vi "PDash - Create DQMH Module Template.vi"(11 "Template Folder":path) -> (0 "error out":errorcluster)   [LabVIEW 2020]
doc: "_____\nCreated using DQMH Event Scripter 7.1.0.1447."
uses:
  PantherDashboard Scripting Hooks/Panther Dasboard Scripting Hooks.lvlib
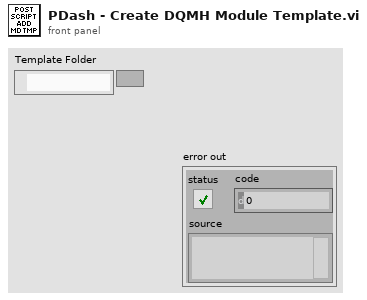
[diagram p1: front panel]
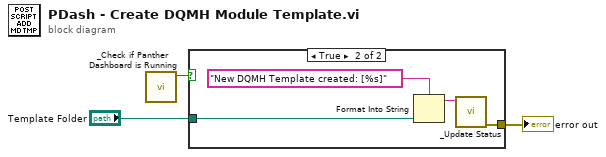
[diagram p0: block diagram]
diagram:
  n1 = call "_Check if Panther Dashboard is Running.vi"() -> ("Panther Dashboard is Running?"=w1:bool)  [unwired: 10 in, 1 out]
  n2 = case shown="True" w1 {
    tunnel: [_ w7] -> w3
    tunnel: "Template Folder" -> [_ w5]
    frame False {
    }
    frame True {
      n3 = Format Into String(format string="New DQMH Template created: [%s]", w5) -> (resulting string=w4:string)  [unwired: 2 in, 1 out]
      n4 = call "_Update Status.vi"("Status"=w4) -> ("error out"=w7:errorcluster)  [unwired: 10 in]
    }
  }
  "error out" <- w3
